vi "Get Enqueuer.vi"(8 "error in (no error)":errorcluster, 11 "View Template in":refnum<class "[V] Waveform.lvclass">) -> (0 "error out":errorcluster, 3 "View Template out":refnum<class "[V] Waveform.lvclass">)   [LabVIEW 2023, in "[V] Waveform.lvlib" / "[V] Waveform.lvclass"]
uses:
  [V] Waveform.lvclass
  [V] Waveform.lvclass/[V] Waveform.ctl
  <vilib>/ActorFramework/Actor/Actor.lvclass
  C:/Program Files (x86)/National Instruments/LabVIEW 2023/vi.lib/ActorFramework/Actor/Actor.lvclass
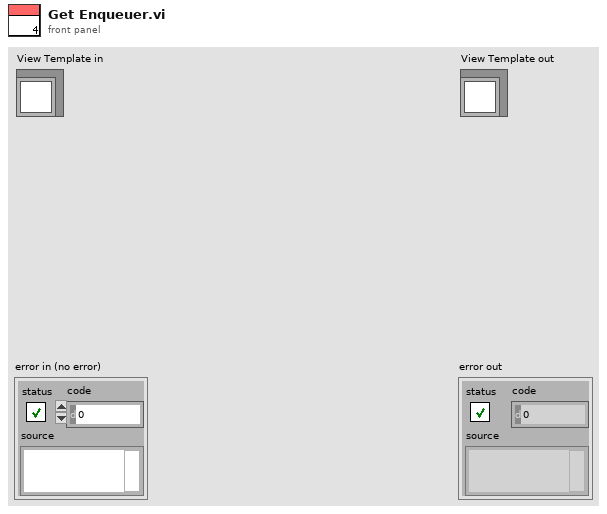
[diagram p1: front panel]
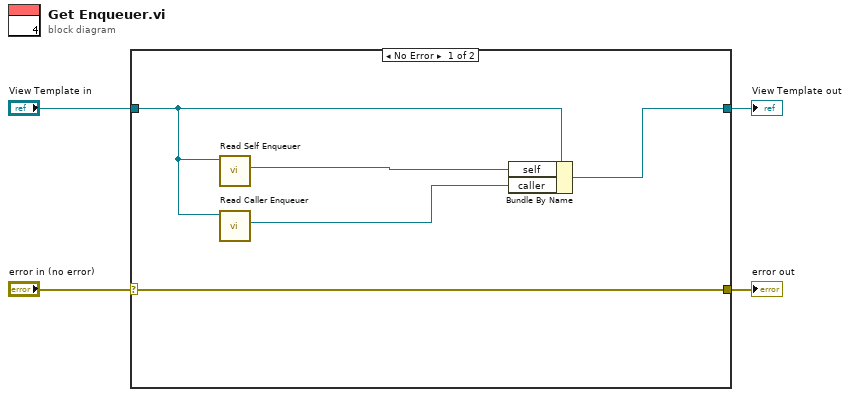
[diagram p0: block diagram]
diagram:
  n1 = case shown="No Error" "error in (no error)" {
    selector: "error in (no error)" -> [w9 w11]
    tunnel: [w9 w11] -> w3
    tunnel: [w5 w10] -> w1
    tunnel: "View Template in" -> [w8 w10]
    frame No Error {
      n2 = call <vilib>:"Read Self Enqueuer.vi"("Actor"=w8) -> ("Self Enqueuer"=w7:refnum<class "Message Enqueuer.lvclass">)  [unwired: 10 in]
      n3 = call <vilib>:"Read Caller Enqueuer.vi"("Actor"=w8) -> ("Caller Enqueuer"=w6:refnum<class "Message Enqueuer.lvclass">)  [unwired: 10 in]
      n4 = Bundle By Name(cluster=w8, "self"=w7, "caller"=w6) -> (w5:refnum<class "[V] Waveform.lvclass">)
    }
    frame Error {
    }
  }
  "error out" <- w3
  "View Template out" <- w1
